vi "Swerve Wheelold.vi"(7 "Wheel":T1(ring), 10 "Inputs":dbl[](array[numeric])) -> (1 "Speed":dbl, 2 "Motor Output":dbl)   [LabVIEW 2018]
uses:
  <vilib>/Rock Robotics/WPI/ThirdParty/Phoenix-LabVIEW/Motor Controller/Controls/CTRE_Phoenix_MotorControl_ControlMode.ctl
  <vilib>/addons/control/pid/pid.llb/PID (DBL).vi
  <vilib>/addons/control/pid/NI_PID_pid.lvlib
panel:
  out "PID Values":cluster{"P":dbl, "I":dbl, "D":dbl}
  # "Swerve Wheel Control\nFRC Team 34"
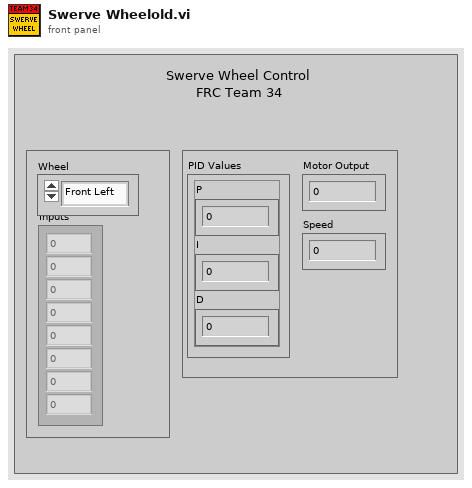
[diagram p1: front panel]
types:
  T1 = enum16{"Front Left", "Front Right", "Back Left", "Back Right"}
  T2 = cluster{"proportional gain (Kc)":dbl, "integral time (Ti, min)":dbl, "derivative time (Td, min)":dbl}
  T3 = enum16{"Z Axis", "Y", "X", "Rot. Point X", "Rot. Point Y", "Width/2", "Max", "Length/2"}
  T4 = typedef "CTRE_Phoenix_MotorControl_ControlMode.ctl" = u16
  T5 = enum16{"Z", "Y", "X", "Rot. Point X", "Rot. Point Y", "Width/2", "Max", "Length/2"}
  T6 = typedef "WPI_MotorControlDeviceRef.ctl" = cluster{"DeviceStatus":errorcluster, "Type":T7, "PWM":cluster{"PWM Channel":T8, "DeadBand":T9}, "CAN":cluster{"Device Number":u8, "SetOutput VI Ref":variant, "GetOutput VI Ref":variant, "Enable VI Ref":variant, "Disable VI Ref":variant, "Data":variant}, "Invert":bool, "DIO PWM":cluster{"PWM \"Enable\" Channel":T8, "DIOChannel":T10, "PWM Rate":dbl}}
  T7 = typedef "WPI_MotorControlType.ctl" = enum16{"PWM", "CAN", "DIO PWM"}
  T8 = typedef "FPGA_DIOPWMChannel.ctl" = enum8{"PWM 0", "PWM 1", "PWM 2", "PWM 3", "PWM 4", "PWM 5", "PWM 6", "PWM 7", "PWM 8", "PWM 9", "PWM MXP 0", "PWM MXP 1", "PWM MXP 2", "PWM MXP 3", "PWM MXP 4", "PWM MXP 5", "PWM MXP 6", "PWM MXP 7", "PWM MXP 8", "PWM MXP 9", "Invalid"}
  T9 = typedef "WPI_PWMDeadband.ctl" = cluster{"Name":string, "maxPositivePwm":i32, "minPositivePwm":i32, "centerPwm":i32, "maxNegativePwm":i32, "minNegativePwm":i32, "angularRange":u16}
  T10 = typedef "FPGA_DIOChannel.ctl" = enum8{"DIO 0", "DIO 1", "DIO 2", "DIO 3", "DIO 4", "DIO 5", "DIO 6", "DIO 7", "DIO 8", "DIO 9", "DIO MXP 0", "DIO MXP 1", "DIO MXP 2", "DIO MXP 3", "DIO MXP 4", "DIO MXP 5", "DIO MXP 6", "DIO MXP 7", "DIO MXP 8", "DIO MXP 9", "DIO MXP 10", "DIO MXP 11", "DIO MXP 12", "DIO MXP 13", "DIO MXP 14", "DIO MXP 15", "SPI Port CS1", "SPI Port CS2", "SPI Port CS3", "SPI Port MISO", "SPI Port MOSI", "Invalid"}
  T11 = typedef "WPI_EncoderDevRef.ctl" = cluster{"DevStatus":errorcluster, "EncoderIndex":T12, "CounterIndex":T13, "DistancePerCount":dbl, "Decoding Type":T14}
  T12 = typedef "FPGA_EncoderIdx.ctl" = enum8{"Enc 0", "Enc 1", "Enc 2", "Enc 3", "Enc 4", "Enc 5", "Enc 6", "Enc 7", "Invalid"}
  T13 = typedef "FPGA_CounterCtrSystemIndex.ctl" = enum8{"Ctr 0", "Ctr 1", "Ctr 2", "Ctr 3", "Ctr 4", "Ctr 5", "Ctr 6", "Ctr 7", "Invalid"}
  T14 = typedef "WPI_EncoderType.ctl" = enum16{"1x", "2x", "4x"}
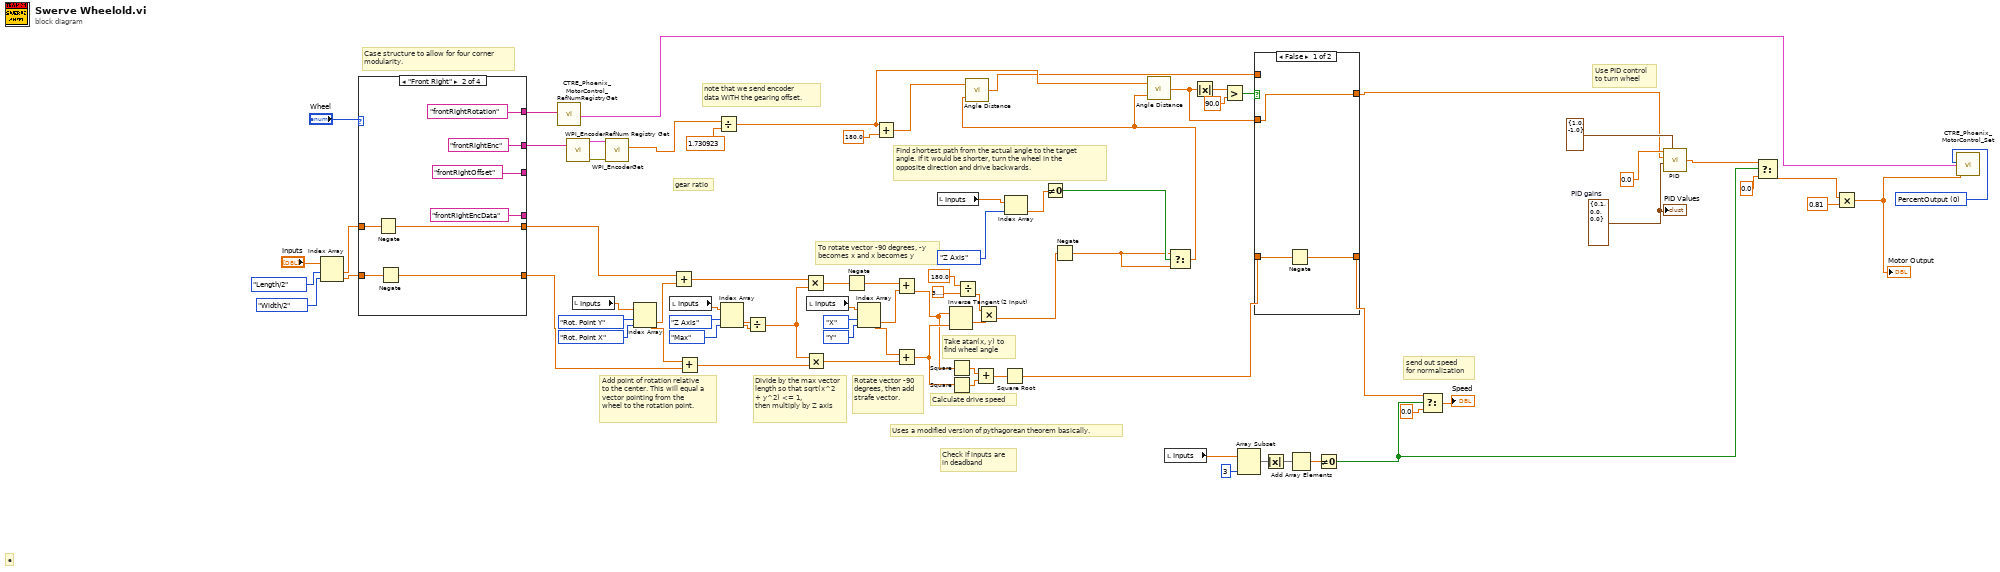
[diagram p0: block diagram]
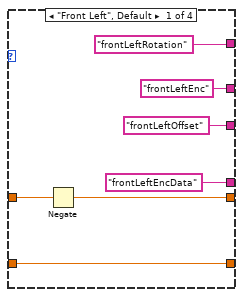
[diagram p3: hidden frame]
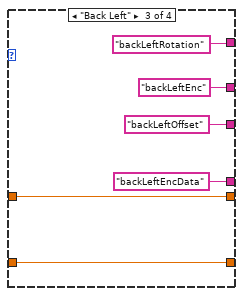
[diagram p4: hidden frame]
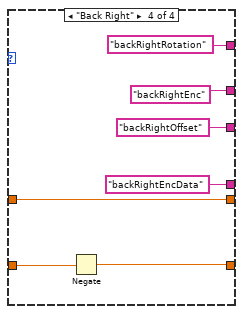
[diagram p5: hidden frame]
diagram:
  w5 = T2 {"proportional gain (Kc)"=0.1, "integral time (Ti, min)"=0.0, "derivative time (Td, min)"=0.0}  # PID gains
  w27 = T4 0 items=["PercentOutput"=0, "Position"=1, "Velocity"=2, "Current"=3, "Follower"=5, "MotionProfile"=6, "MotionMagic"=7, "MotionMagicArc"=8, "MotionProfileArc"=10, "Disabled"=15] ("Control Mode")
  # "gear ratio"
  # "Uses a modified version of pythagorean theorem basically."
  # "e"
  # "note that we send encoder \ndata WITH the gearing offset."
  # "Case structure to allow for four corner\nmodularity."
  # "To rotate vector -90 degrees, -y becomes x and x becomes y"
  # "send out speed\nfor normalization"
  # "Use PID control\nto turn wheel"
  # "Find shortest path from the actual angle to the target angle. If it would be shorter, turn the wheel in the opposite direction and drive backwards."
  # "Divide by the max vector length so that sqrt(x^2 + y^2) <= 1,\nthen multiply by Z axis"
  # "Add point of rotation relative to the center. This will equal a vector pointing from the\nwheel to the rotation point."
  # "Check if inputs are\nin deadband"
  # "Take atan(x, y) to find wheel angle"
  # "Calculate drive speed"
  # "Rotate vector -90 degrees, then add strafe vector."
  n1 = Index Array(array="Inputs", index #1=T5."Length/2", index #2=T5."Width/2") -> (element #1=w76:dbl, element #2=w75:dbl)
  n2 = case shown="\"Front Right\"" "Wheel" {
    tunnel: w76 -> [w87 w95 w101 w108]
    tunnel: w75 -> [w85 w93 w100 w107]
    tunnel: [w86 w94 w101 w108] -> w1
    tunnel: [w85 w92 w100 w106] -> w49
    tunnel: ["frontLeftRotation" "frontRightRotation" "backLeftRotation" "backRightRotation"] -> w29
    tunnel: ["frontLeftEnc" ("refnum name") "frontRightEnc" ("refnum name") "backLeftEnc" ("refnum name") "backRightEnc" ("refnum name")] -> w57
    tunnel: ["frontLeftOffset" ("Name") "frontRightOffset" ("Name") "backLeftOffset" ("Name") "backRightOffset" ("Name")] -> _
    tunnel: ["frontLeftEncData" ("Name") "frontRightEncData" ("Name") "backLeftEncData" ("Name") "backRightEncData" ("Name")] -> _
    frame "Front Left", Default {
      n3 = Negate(x=w87) -> (-x=w86:dbl)
    }
    frame "Front Right" {
      n4 = Negate(x=w95) -> (-x=w94:dbl)
      n5 = Negate(x=w93) -> (-x=w92:dbl)
    }
    frame "Back Left" {
    }
    frame "Back Right" {
      n6 = Negate(x=w107) -> (-x=w106:dbl)
    }
  }
  n7 = call <vilib>:"CTRE_Phoenix_MotorControl_RefNumRegistryGet.vi"("refnum name"=w29) -> ("PhoenixMotorControlDevRef"=w28:T6)  [unwired: 9 in, 1 out]
  n8 = call <vilib>:"WPI_EncoderRefNum Registry Get.vi"("refnum name"=w57) -> ("error out"=w56:errorcluster, "EncoderDevRef"=w55:T11)  [unwired: 9 in]
  n9 = local read "Inputs"() -> (w52:dbl[])
  n10 = call <vilib>:"WPI_EncoderGet.vi"("error in (no error)"=w56, "EncoderDevRef"=w55) -> ("Distance"=w2:dbl)  [unwired: 4 in, 5 out]
  n11 = Index Array(array=w52, index #1=T5."Rot. Point Y", index #2=T5."Rot. Point X") -> (element #1=w50:dbl, element #2=w51:dbl)
  n12 = local read "Inputs"() -> (w58:dbl[])
  n13 = Add(x=w1, y=w50) -> (x+y=w48:dbl)
  n14 = Add(x=w51, y=w49) -> (x+y=w67:dbl)
  n15 = Divide(x=w2, y=1.730923) -> (x/y=w25:dbl)
  n16 = Index Array(array=w58, index #1=T3."Z Axis", index #2=T5."Max") -> (element #1=w32:dbl, element #2=w31:dbl)
  n17 = Divide(x=w32, y=w31) -> (x/y=w16:dbl)
  n18 = Multiply(x=w48, y=w16) -> (x*y=w60:dbl)
  n19 = Multiply(x=w16, y=w67) -> (x*y=w63:dbl)
  n20 = local read "Inputs"() -> (w35:dbl[])
  n21 = Negate(x=w60) -> (-x=w59:dbl)
  n22 = Index Array(array=w35, index #1=T5."X", index #2=T5."Y") -> (element #1=w34:dbl, element #2=w33:dbl)
  n23 = Add(x=w25, y=180.0) -> (x+y=w24:dbl)
  n24 = Add(x=w59, y=w34) -> (x+y=w61:dbl)
  n25 = Add(x=w33, y=w63) -> (x+y=w62:dbl)
  n26 = local read "Inputs"() -> (w14:dbl[])
  n27 = Inverse Tangent (2 Input)(1:w62, 2:w61) -> (0:w74:dbl)
  n28 = Square(x=w61) -> (x^2=w64:dbl)
  n29 = Square(x=w62) -> (x^2=w73:dbl)
  n30 = Divide(x=180.0 ("y"), y=3.141592653589793) -> (x/y=w71:dbl)
  n31 = Add(x=w64, y=w73) -> (x+y=w72:dbl)
  n32 = Multiply(x=w71, y=w74) -> (x*y=w10:dbl)
  n33 = Square Root(x=w72) -> (sqrt(x)=w22:dbl)
  n34 = Index Array(array=w14, index=T3."Z Axis") -> (element=w12:dbl)
  n35 = Not Equal To 0?(x=w12) -> (x != 0?=w11:bool)
  n36 = Negate(x=w10) -> (-x=w6:dbl)
  n37 = local read "Inputs"() -> (w43:dbl[])
  n38 = Select(t=w6, s=w11, f=w6) -> (s? t:f=w15:dbl)
  n39 = call "Angle Distance.vi"("Target Angle"=w15, "Current Angle"=w24) -> ("Distance"=w23:dbl)
  n40 = call "Angle Distance.vi"("Target Angle"=w15, "Current Angle"=w25) -> ("Distance"=w19:dbl)
  n41 = Absolute Value(x=w19) -> (abs(x)=w18:dbl)
  n42 = Greater?(x=w18, y=90.0) -> (0:w20:bool)
  n43 = Array Subset(array=w43, length=3) -> (w45:dbl[])  [unwired: 1 in]
  n44 = case shown="False" w20 {
    tunnel: w22 -> [w110 w112]
    tunnel: w19 -> [w111 _]
    tunnel: w23 -> [_ w113]
    tunnel: [w109 w112] -> w21
    tunnel: [w111 w113] -> w3
    frame False {
      n45 = Negate(x=w110) -> (-x=w109:dbl)
    }
    frame True {
    }
  }
  n46 = Absolute Value(x=w45) -> (abs(x)=w44:dbl[])
  n47 = Add Array Elements(numeric array=w44) -> (sum=w46:dbl)
  n48 = Not Equal To 0?(x=w46) -> (x != 0?=w36:bool)
  n49 = Select(t=w21, s=w36, f=0.0) -> (s? t:f=→"Speed":dbl)
  n50 = call-poly <vilib>:"PID.vi"("output range"=cluster{"output high":dbl, "output low":dbl} {"output high"=1.0, "output low"=-1.0}, "PID gains"=w5, "process variable"=w3, "setpoint"=0.0) -> ("output"=w38:dbl)  [unwired: 6 in, 1 out]
  n51 = Select(t=w38, s=w36, f=0.0) -> (s? t:f=w9:dbl)
  n52 = Multiply(x=w9, y=0.81) -> (x*y=w7:dbl)
  "Motor Output" <- w7
  n53 = call <vilib>:"CTRE_Phoenix_MotorControl_Set.vi"("Output"=w7, "Control Mode"=w27, "PhoenixMotorControlDevRef"=w28) -> ()  [unwired: 7 in, 2 out]
  "PID Values" <- w5
